vi "表面处理文件夹选择.vi"(8 "error in (no error)":errorcluster caption="错误输入（无错误）", 10 "前后位置":string(combo), 11 "CCD":string(combo)) -> (0 "error out":errorcluster caption="错误输出", 2 "All Files in Dir":path[](array[path]) caption="目录中的所有文件", 3 "文件个数显示":i32)   [LabVIEW 2017]
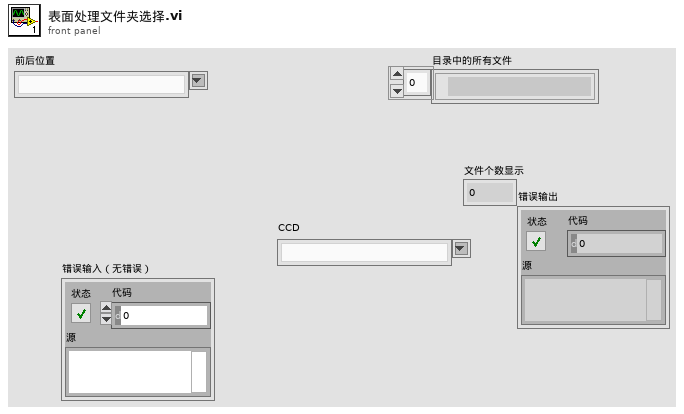
[diagram p1: front panel]
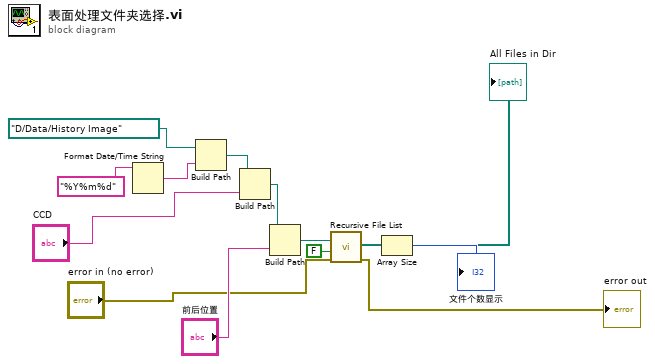
[diagram p0: block diagram]
diagram:
  n1 = Format Date/Time String(time format string (%c)="%Y%m%d" ("时间格式字符串(%c)")) -> (date/time string=w9:string)  [unwired: 2 in]
  n2 = Build Path(base path=path "D:/Data/History Image" ("基路径"), name or relative path=w9) -> (appended path=w11:path)
  n3 = Build Path(base path=w11, name or relative path="CCD") -> (appended path=w10:path)
  n4 = Build Path(base path=w10, name or relative path="前后位置") -> (appended path=w8:path)
  n5 = call <vilib>:"Recursive File List.vi"("error in (no error)"="error in (no error)", "Continue Recursing on Error? (F)"=FALSE, "Folder Path"=w8) -> ("error out"=→"error out":errorcluster, "All Files in Dir"=w6:path[])  [unwired: 4 in, 3 out]
  "All Files in Dir" <- w6
  n6 = Array Size(array=w6) -> (size(s)=→"文件个数显示":i32)
